vi "Recurse.vi"(6 "Teller":refnum<class "Teller.lvclass">, 7 "Actor in":refnum<class "Actor.lvclass">, 9 "Parent Stopped":bool, 10 "Safe Stop":bool=TRUE) -> (0 "Error out":errorcluster, 5 "Actor out":refnum<class "Actor.lvclass">)   [LabVIEW 2025, in "jettl.lvlib" / "Stop Msg.lvlib"]
uses:
  Stop Msg.lvlib
  Actor/Actor.lvclass
  Teller/Teller/Teller.lvclass
  Stop Msg/Stop Msg.lvclass
  jettl.lvlib
  Stop Msg Output/Stop Msg Output.lvclass
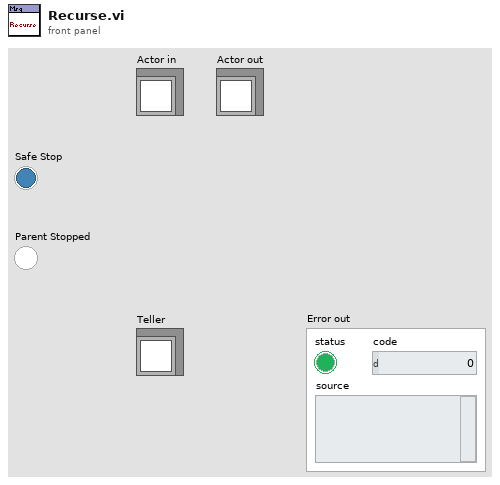
[diagram p1: front panel]
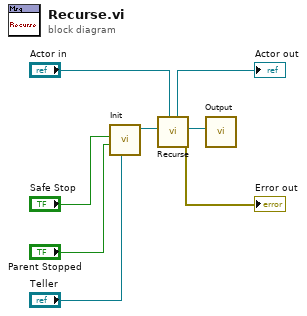
[diagram p0: block diagram]
diagram:
  n1 = call "Init.vi"("Teller"="Teller", "Parent Stopped"="Parent Stopped", "Safe Stop"="Safe Stop") -> ("Stop Msg out"=w3:refnum<class "Stop Msg.lvclass">)  [unwired: 8 in]
  n2 = call "Recurse.vi"("Actor in"="Actor in", "Msg"=w3) -> ("Error out"=→"Error out":errorcluster, "Msg Output"=w2:refnum<class "Msg Output.lvclass">, "Actor out"=→"Actor out":refnum<class "Actor.lvclass">)  [unwired: 7 in]
  n3 = call "Output.vi"("Msg Output"=w2) -> ()  [unwired: 11 in]
